vi "From bytes.vi"(8 "error in (no error)":errorcluster, 11 "Bytes":u8[](array[numeric]) format="%x") -> (0 "error out":errorcluster, 1 "remaining bytes":u8[](array[numeric]), 3 "MessagePackNumeric out":refnum<class "MessagePackNumeric.lvclass">, 5 "Type":T1)   [LabVIEW 2020, in "MessagePack.lvlib" / "MessagePackNumeric.lvclass"]
uses:
  MessagePackNumeric.lvclass
  MsgPack Object Types.ctl
  Object Family.ctl
  MessagePackNumeric.lvclass/MessagePackNumeric.ctl
  <vilib>/Utility/error.llb/Error Cluster From Error Code.vi
  <vilib>/ErrorRing/Error Ring.xnode
  MessagePack.lvclass
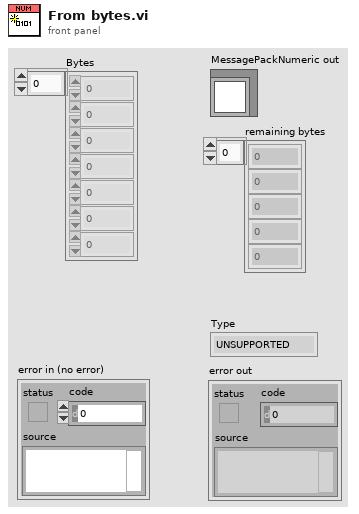
[diagram p1: front panel]
types:
  T1 = typedef "MessagePack.lvlib/MessagePack.lvclass/MsgPack Object Types.ctl" = enum16{"UNSUPPORTED", "POSINT", "NEGINT", "FIXMAP", "FIXARRAY", "FIXSTR", "NIL", "FALSE", "TRUE", "BIN8", "BIN16", "BIN32", "EXT8", "EXT16", "EXT32", "FLOAT32", "FLOAT64", "UINT8", "UINT16", "UINT32", "UINT64", "INT8", "INT16", "INT32", "INT64", "FIXEXT1", "FIXEXT2", "FIXEXT4", "FIXEXT8", "FIXEXT16", "STR8", "STR16", "STR32", "ARRAY16", "ARRAY32", "MAP16", "MAP32"}
  T2 = typedef "MessagePack.lvlib/MessagePack.lvclass/Object Family.ctl" = enum16{"Unsupported", "Nil", "Numeric", "Array", "Map", "String", "Binary", "Boolean", "Ext"}
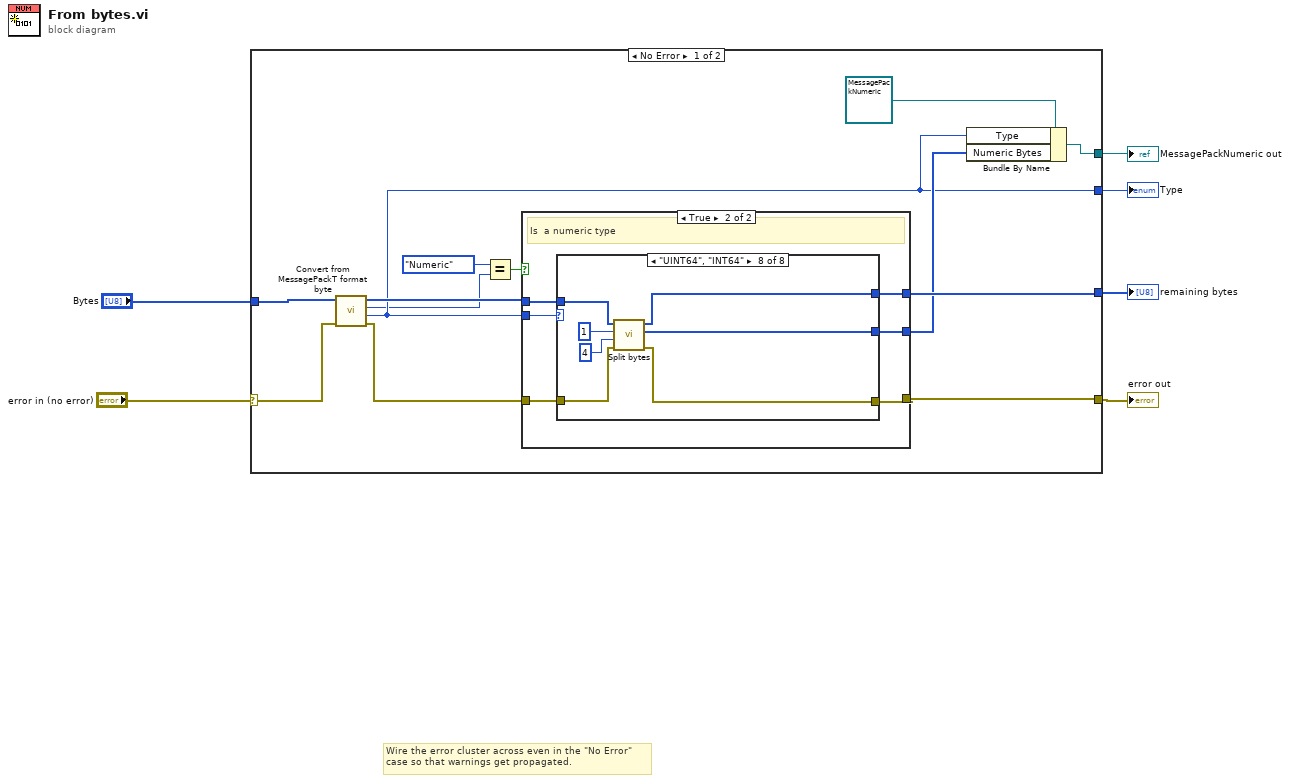
[diagram p0: block diagram]
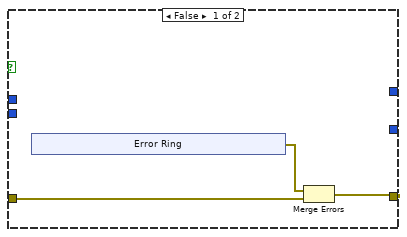
[diagram p2: hidden frame]
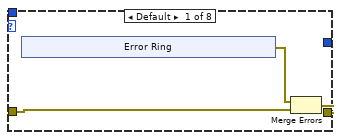
[diagram p3: hidden frame]
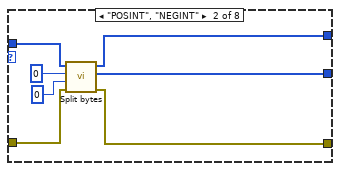
[diagram p4: hidden frame]
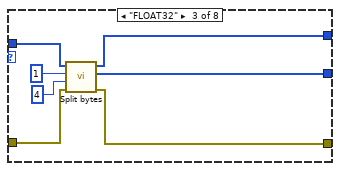
[diagram p5: hidden frame]
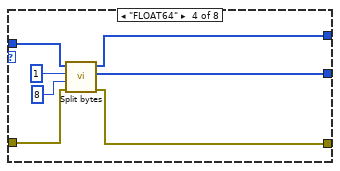
[diagram p6: hidden frame]
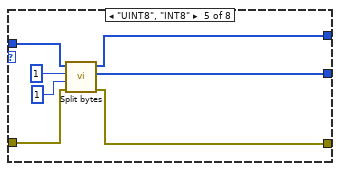
[diagram p7: hidden frame]
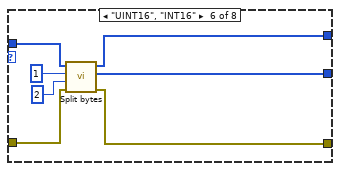
[diagram p8: hidden frame]
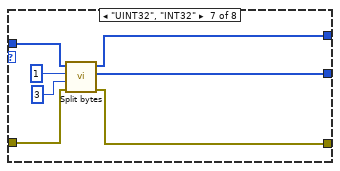
[diagram p9: hidden frame]
diagram:
  # "Wire the error cluster across even in the \"No Error\"\ncase so that warnings get propagated."
  n1 = case shown="No Error" "error in (no error)" {
    selector: "error in (no error)" -> [w19 w89]
    tunnel: [w17 w89] -> w5
    tunnel: "Bytes" -> [w11 _]
    tunnel: [w15 _] -> w3
    tunnel: [w9 _] -> w2
    tunnel: [w12 _] -> w1
    frame No Error {
      n2 = call "Convert from MessagePackT format byte.vi"("error in (no error)"=w19, "Bytes in"=w11) -> ("error out"=w16:errorcluster, "MsgPack Type"=w9:T1, "Object Family Type"=w8:T2, "Bytes out"=w10:u8[])  [unwired: 6 in]
      n3 = Equal?(x=Object_Family."Numeric", y=w8) -> (x = y?=w18:bool)
      n4 = case shown="True" w18 {
        tunnel: [w21 w28] -> w17
        tunnel: w16 -> [w20 w29]
        tunnel: w9 -> [_ w32]
        tunnel: w10 -> [_ w31]
        tunnel: [_ w30] -> w15
        tunnel: [_ w27] -> w13
        frame False {
          n5 = xnode "Error Ring"() -> ("error out"=w22:errorcluster)
          n6 = Merge Errors(w22, w20) -> (w21:errorcluster)
        }
        frame True {
          # "Is  a numeric type"
          n7 = case shown="\"UINT64\", \"INT64\"" w32 {
            tunnel: w31 -> [_ w46 w53 w60 w67 w74 w81 w88]
            tunnel: [_ w43 w50 w57 w64 w71 w78 w85] -> w30
            tunnel: w29 -> [w33 w42 w49 w56 w63 w70 w77 w84]
            tunnel: [w34 w41 w48 w55 w62 w69 w76 w83] -> w28
            tunnel: [_ w40 w47 w54 w61 w68 w75 w82] -> w27
            frame Default {
              n8 = xnode "Error Ring"() -> ("error out"=w35:errorcluster)
              n9 = Merge Errors(w35, w33) -> (w34:errorcluster)
            }
            frame "POSINT", "NEGINT" {
              n10 = call "Split bytes.vi"("error in"=w42, "End index"=0, "Start index"=0, "bytes in"=w46) -> ("error out"=w41:errorcluster, "selected bytes"=w40:u8[], "remaining bytes"=w43:u8[])  [unwired: 4 in, 1 out]
            }
            frame "FLOAT32" {
              n11 = call "Split bytes.vi"("error in"=w49, "End index"=4, "Start index"=1, "bytes in"=w53) -> ("error out"=w48:errorcluster, "selected bytes"=w47:u8[], "remaining bytes"=w50:u8[])  [unwired: 4 in, 1 out]
            }
            frame "FLOAT64" {
              n12 = call "Split bytes.vi"("error in"=w56, "End index"=8, "Start index"=1, "bytes in"=w60) -> ("error out"=w55:errorcluster, "selected bytes"=w54:u8[], "remaining bytes"=w57:u8[])  [unwired: 4 in, 1 out]
            }
            frame "UINT8", "INT8" {
              n13 = call "Split bytes.vi"("error in"=w63, "End index"=1, "Start index"=1, "bytes in"=w67) -> ("error out"=w62:errorcluster, "selected bytes"=w61:u8[], "remaining bytes"=w64:u8[])  [unwired: 4 in, 1 out]
            }
            frame "UINT16", "INT16" {
              n14 = call "Split bytes.vi"("error in"=w70, "End index"=2, "Start index"=1, "bytes in"=w74) -> ("error out"=w69:errorcluster, "selected bytes"=w68:u8[], "remaining bytes"=w71:u8[])  [unwired: 4 in, 1 out]
            }
            frame "UINT32", "INT32" {
              n15 = call "Split bytes.vi"("error in"=w77, "End index"=3, "Start index"=1, "bytes in"=w81) -> ("error out"=w76:errorcluster, "selected bytes"=w75:u8[], "remaining bytes"=w78:u8[])  [unwired: 4 in, 1 out]
            }
            frame "UINT64", "INT64" {
              n16 = call "Split bytes.vi"("error in"=w84, "End index"=4, "Start index"=1, "bytes in"=w88) -> ("error out"=w83:errorcluster, "selected bytes"=w82:u8[], "remaining bytes"=w85:u8[])  [unwired: 4 in, 1 out]
            }
          }
        }
      }
      n17 = Bundle By Name(cluster=refnum<class "MessagePackNumeric.lvclass"> refnum ("MessagePack.lvlib:MessagePackNumeric.lvclass"), "Type"=w9, "Numeric Bytes"=w13) -> (w12:refnum<class "MessagePackNumeric.lvclass">)
    }
    frame Error {
    }
  }
  "error out" <- w5
  "MessagePackNumeric out" <- w1
  "remaining bytes" <- w3
  "Type" <- w2
